vi "Close.vi"(8 "Error In":errorcluster, 11 "Adept Config":T1) -> (0 "Error Out":errorcluster)   [LabVIEW 2011, in "LVH-Adept.lvlib"]
doc: "Close the connection to a Digilent FPGA board."
uses:
  LVH-Adept.lvlib
  Private/Type Defs/Device Config.ctl
  Private/Type Defs/Status.ctl
  Private/DMGR/DMGR.lvlib
  Private/DEPP/DEPP.lvlib
  Private/DJTG/DJTG.lvlib
  Private/DSTM/DSTM.lvlib
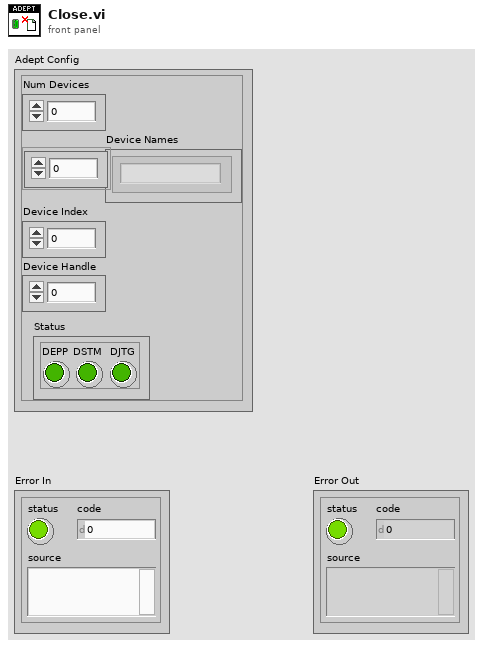
[diagram p1: front panel]
types:
  T1 = typedef "LVH-Adept.lvlib/Device Config.ctl" = cluster{"Num Devices":i32, "Device Names":string[], "Device Index":u16, "Device Handle":u32, "Status":T2}
  T2 = typedef "LVH-Adept.lvlib/Status.ctl" = cluster{"DEPP":bool, "DSTM":bool, "DJTG":bool}
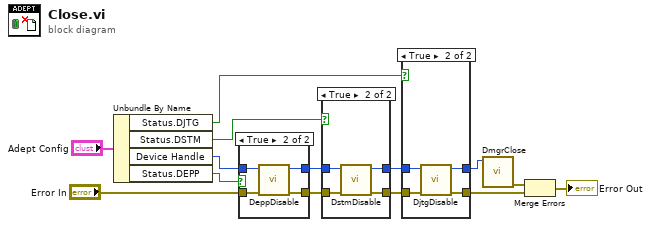
[diagram p0: block diagram]
diagram:
  n1 = Unbundle By Name("Adept Config") -> ("Status.DJTG"=w2:bool, "Status.DSTM"=w1:bool, "Device Handle"=w9:u32, "Status.DEPP"=w12:bool)
  n2 = case shown="True" w12 {
    tunnel: "Error In" -> [w16 w20]
    tunnel: [w16 w19] -> w10
    tunnel: w9 -> [w15 w18]
    tunnel: [w15 w17] -> w5
    frame False {
    }
    frame True {
      n3 = call "DeppDisable.vi"("Error In"=w20, "Device Handle"=w18) -> ("Error Out"=w19:errorcluster, "Device Handle"=w17:u32)  [unwired: 8 in]
    }
  }
  n4 = case shown="True" w1 {
    tunnel: w10 -> [w22 w26]
    tunnel: [w22 w25] -> w8
    tunnel: w5 -> [w21 w24]
    tunnel: [w21 w23] -> w4
    frame False {
    }
    frame True {
      n5 = call "DstmDisable.vi"("Error In"=w26, "Device Handle"=w24) -> ("Error Out"=w25:errorcluster, "Device Handle"=w23:u32)  [unwired: 8 in]
    }
  }
  n6 = case shown="True" w2 {
    tunnel: w8 -> [w28 w32]
    tunnel: [w28 w31] -> w6
    tunnel: w4 -> [w27 w30]
    tunnel: [w27 w29] -> w3
    frame False {
    }
    frame True {
      n7 = call "DjtgDisable.vi"("Error In"=w32, "Device Number"=w30) -> ("Error Out"=w31:errorcluster, "Device Number"=w29:u32)  [unwired: 8 in]
    }
  }
  n8 = call "DmgrClose.vi"("hif"=w3) -> ("Error Out"=w14:errorcluster)  [unwired: 10 in]
  n9 = Merge Errors(w14, w6) -> (→"Error Out":errorcluster)
